vi "Del_First_And_last.vi"(11 "Array in":dbl[](array[numeric])) -> (3 "Array out":dbl[](array[numeric]))   [LabVIEW 2020]
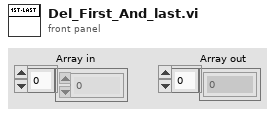
[diagram p1: front panel]
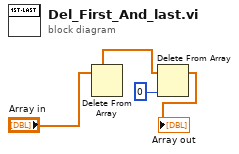
[diagram p0: block diagram]
diagram:
  n1 = Delete From Array(array="Array in") -> (array with subset deleted=w2:dbl[])  [unwired: 2 in, 1 out]
  n2 = Delete From Array(array=w2, index=0) -> (array with subset deleted=→"Array out":dbl[])  [unwired: 1 in, 1 out]
